vi "CANOpen_Send SDOs from list.vi"(6 "SDO queues":T1, 7 "Nodes":T4[](array[typedef]) {"NMT"."Node init static SDO state" items=["start remote node"=1, "enter pre-operational"=128]; "NMT"."Node run state" items=["start remote node"=1, "stop remote node"=2, "enter pre-operational"=128, "reset node"=129, "reset communication"=130]; "Dynamic SDOs"."Sub-Index (0)" format="%.0x"; "Dynamic SDOs"."Object Index" format="%.0x"; "Dynamic SDOs"."Block Data" format="%.0x"; "RPDOs"."PDO Channel" items=["PDO 1", "PDO 2", "PDO 3", "PDO 4"]; "RPDOs"."Parameters"."Bit Offset" max=8 step=1; "RPDOs"."Parameters"."Byte Offset" max=8 step=1; "TPDOs"."PDO Channel" items=["PDO 1", "PDO 2", "PDO 3", "PDO 4"]; "TPDOs"."Parameters"."Bit Offset" max=8 step=1; "TPDOs"."Parameters"."Byte Offset" max=8 step=1; "SDOs"."Sub-Index (0)" format="%.0x"; "SDOs"."Object Index" format="%.0x"; "SDOs"."Block Data" format="%.0x"}, 8 "error in":errorcluster, 10 "SDO Asynch":T2 {"HW Dyn Read"."Resp Chan."."Chan Refs" format="%.0x"; "HW Dyn Read"."Req Chan."."Chan Refs" format="%.0x"; "HW Dyn Write"."Resp Chan."."Chan Refs" format="%.0x"; "HW Dyn Write"."Req Chan."."Chan Refs" format="%.0x"; "List SDO"."Resp Chan."."Chan Refs" format="%.0x"; "List SDO"."Req Chan."."Chan Refs" format="%.0x"}, 11 "interface object":refnum<k20>) -> (0 "error out":errorcluster, 3 "interface object out":refnum<k20>)   [LabVIEW 2013, in "CANOpen Addon Custom Device.lvlib"]
uses:
  CANOpen Addon Custom Device.lvlib
  CANOpen_Node Message Settings.ctl
  Shared Code/CANOpen_PDO Settings.ctl
  Shared Code/CANOpen_PDO Parameter Settings.ctl
  Shared Code/CANOpen_PDO Data Type.ctl
  System Explorer/SubVIs/CANopen Byte Order.ctl
  Shared Code/CANOpen_SDO Settings.ctl
  CANOpen_NMT Settings.ctl
  Async VIs/CANOpen_Main/SubVIs/CanOpen_NMT_Config.ctl
  Async VIs/CANOpen_Main/SubVIs/CanOpen_NMT_Static detect.ctl
  CANOpen_VS SDOs Data Refs.ctl
  <vilib>/NI Veristand/Custom Device API/Data Reference.ctl
  Async VIs/CANOpen_Main/SubVIs/CanOpen_SDO Dynamic queue.ctl
  Shared Code/CANOpen_SDO queue W data.ctl
  Shared Code/CANOpen_SDO queue mode.ctl
  Shared Code/CANOpen_PDO Data Type in queue.ctl
  Async VIs/CANOpen_Main/SubVIs/CanOpen_SDO queue ref.ctl
  Async VIs/CANOpen_Main/SubVIs/SDO queue.ctl
  <vilib>/NI Veristand/Custom Device Tools/Custom Device Utility Library/RT Debug String Color Spec.ctl
  <vilib>/NI Veristand/Custom Device Tools/Custom Device Utility Library/Custom Device Utility Library.lvlib
  <vilib>/NI Veristand/Custom Device API/Custom Device API.lvlib
panel:
  # "LSB"
  # "MSB"
  # "LSB"
  # "MSB"
  # "LSB"
  # "MSB"
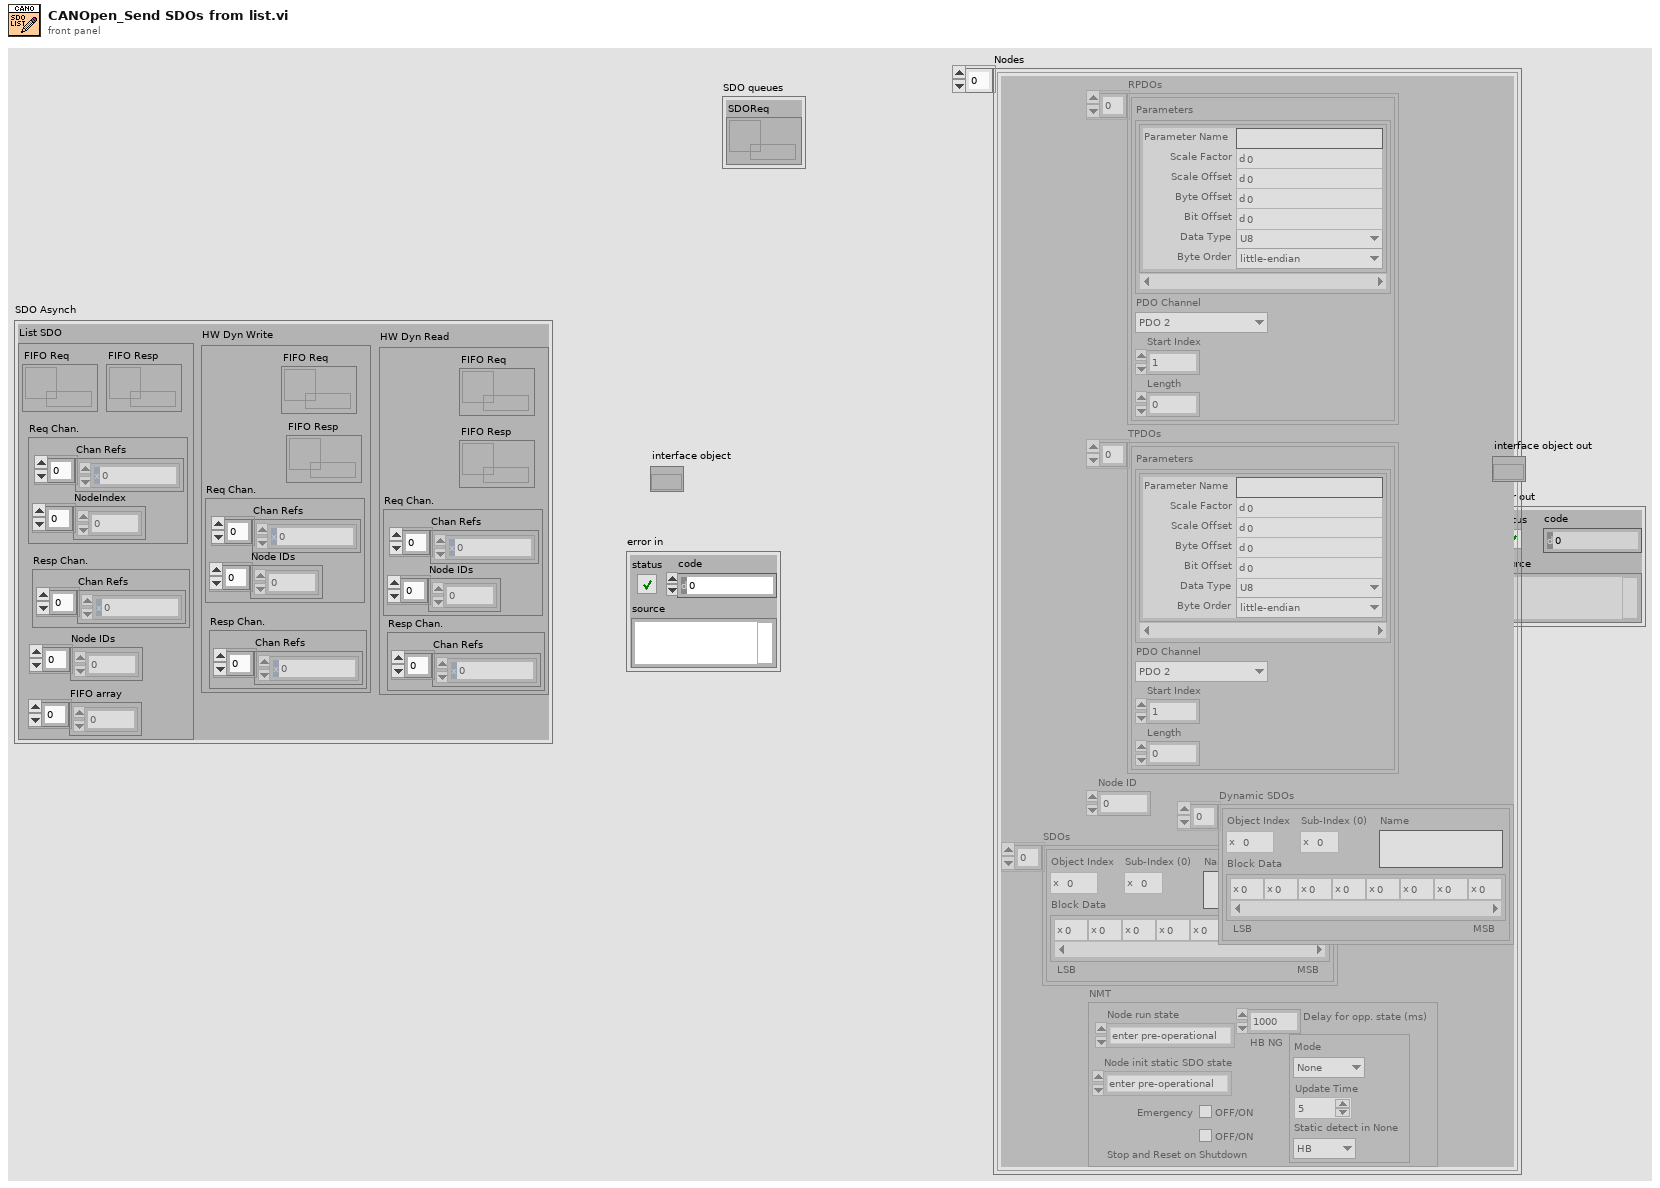
[diagram p1: front panel]
types:
  T1 = typedef "CANOpen Addon Custom Device.lvlib/CanOpen_SDO queue ref.ctl" = cluster{"SDOReq":refnum<queue>}
  T2 = typedef "CANOpen Addon Custom Device.lvlib/CANOpen_VS SDOs Data Refs.ctl" = cluster{"List SDO":cluster{"FIFO Req":refnum<k33>, "Req Chan.":cluster{"Chan Refs":T3[], "NodeIndex":dbl[]}, "FIFO Resp":refnum<k33>, "Resp Chan.":cluster{"Chan Refs":T3[]}, "Node IDs":u8[], "FIFO array":dbl[]}, "HW Dyn Write":cluster{"FIFO Req":refnum<k33>, "FIFO Resp":refnum<k33>, "Req Chan.":cluster{"Chan Refs":T3[], "Node IDs":u8[]}, "Resp Chan.":cluster{"Chan Refs":T3[]}}, "HW Dyn Read":cluster{"FIFO Req":refnum<k33>, "FIFO Resp":refnum<k33>, "Req Chan.":cluster{"Chan Refs":T3[], "Node IDs":u8[]}, "Resp Chan.":cluster{"Chan Refs":T3[]}}}
  T3 = typedef "Custom Device API.lvlib/Data Reference.ctl" = i32
  T4 = typedef "CANOpen_Node Message Settings.ctl" = cluster{"RPDOs":T5[], "TPDOs":T5[], "Node ID":u8, "SDOs":T9[], "Dynamic SDOs":T9[], "NMT":T10}
  T5 = typedef "CANOpen Addon Custom Device.lvlib/CANOpen_PDO Settings.ctl" = cluster{"Parameters":T6[], "PDO Channel":u8, "Start Index":u32, "Length":u32}
  T6 = typedef "CANOpen Addon Custom Device.lvlib/CANOpen_PDO Parameter Settings.ctl" = cluster{"Parameter Name":string, "Scale Factor":dbl, "Scale Offset":dbl, "Byte Offset":u8, "Bit Offset":u8, "Data Type":T7, "Byte Order":T8}
  T7 = typedef "CANOpen Addon Custom Device.lvlib/CANOpen_PDO Data Type.ctl" = enum16{"U8", "U16", "U32", "I8", "I16", "I32", "Single", "Double", "Boolean"}
  T8 = typedef "CANOpen Addon Custom Device.lvlib/CANopen Byte Order.ctl" = enum16{"big-endian network order", "little-endian"}
  T9 = typedef "CANOpen Addon Custom Device.lvlib/CANOpen_SDO Settings.ctl" = cluster{"Object Index":u16, "Sub-Index (0)":u8, "Block Data":u8[], "Name":string}
  T10 = typedef "CANOpen Addon Custom Device.lvlib/CANOpen_NMT Settings.ctl" = cluster{"Node run state":u16, "Emergency":bool, "HB NG":T11, "Delay for opp. state (ms)":dbl, "Node init static SDO state":u16, "Stop and Reset on Shutdown":bool}
  T11 = typedef "CANOpen Addon Custom Device.lvlib/CanOpen_NMT_Config.ctl" = cluster{"Mode":T12, "Update Time":u16, "Static detect in None":T12}
  T12 = typedef "CANOpen Addon Custom Device.lvlib/CanOpen_NMT_Static detect.ctl" = enum16{"None", "HB", "NG"}
  T13 = typedef "CANOpen Addon Custom Device.lvlib/CanOpen_SDO Dynamic queue.ctl" = cluster{"Node ID":u8, "Data":T14}
  T14 = typedef "CANOpen Addon Custom Device.lvlib/CANOpen_SDO queue W data.ctl" = cluster{"Object Index":u16, "Object Sub-Index (0)":u8, "Mode":T15, "Data Type":T16, "Value":dbl, "Status code":dbl, "Byte Order":enum16{"big-endian, network order", "little-endian"}}
  T15 = typedef "CANOpen Addon Custom Device.lvlib/CANOpen_SDO queue mode.ctl" = enum16{"WRITE write", "WRITE response", "READ write", "READ response"}
  T16 = typedef "CANOpen Addon Custom Device.lvlib/CANOpen_PDO Data Type in queue.ctl" = enum16{"U8", "U16", "U32", "I8", "I16", "I32", "Single", "Double"}
  T17 = typedef "CANOpen Addon Custom Device.lvlib/SDO queue.ctl" = cluster{"element":T9, "Node ID":u8}
  T18 = typedef "Custom Device Utility Library.lvlib/RT Debug String Color Spec.ctl" = u16
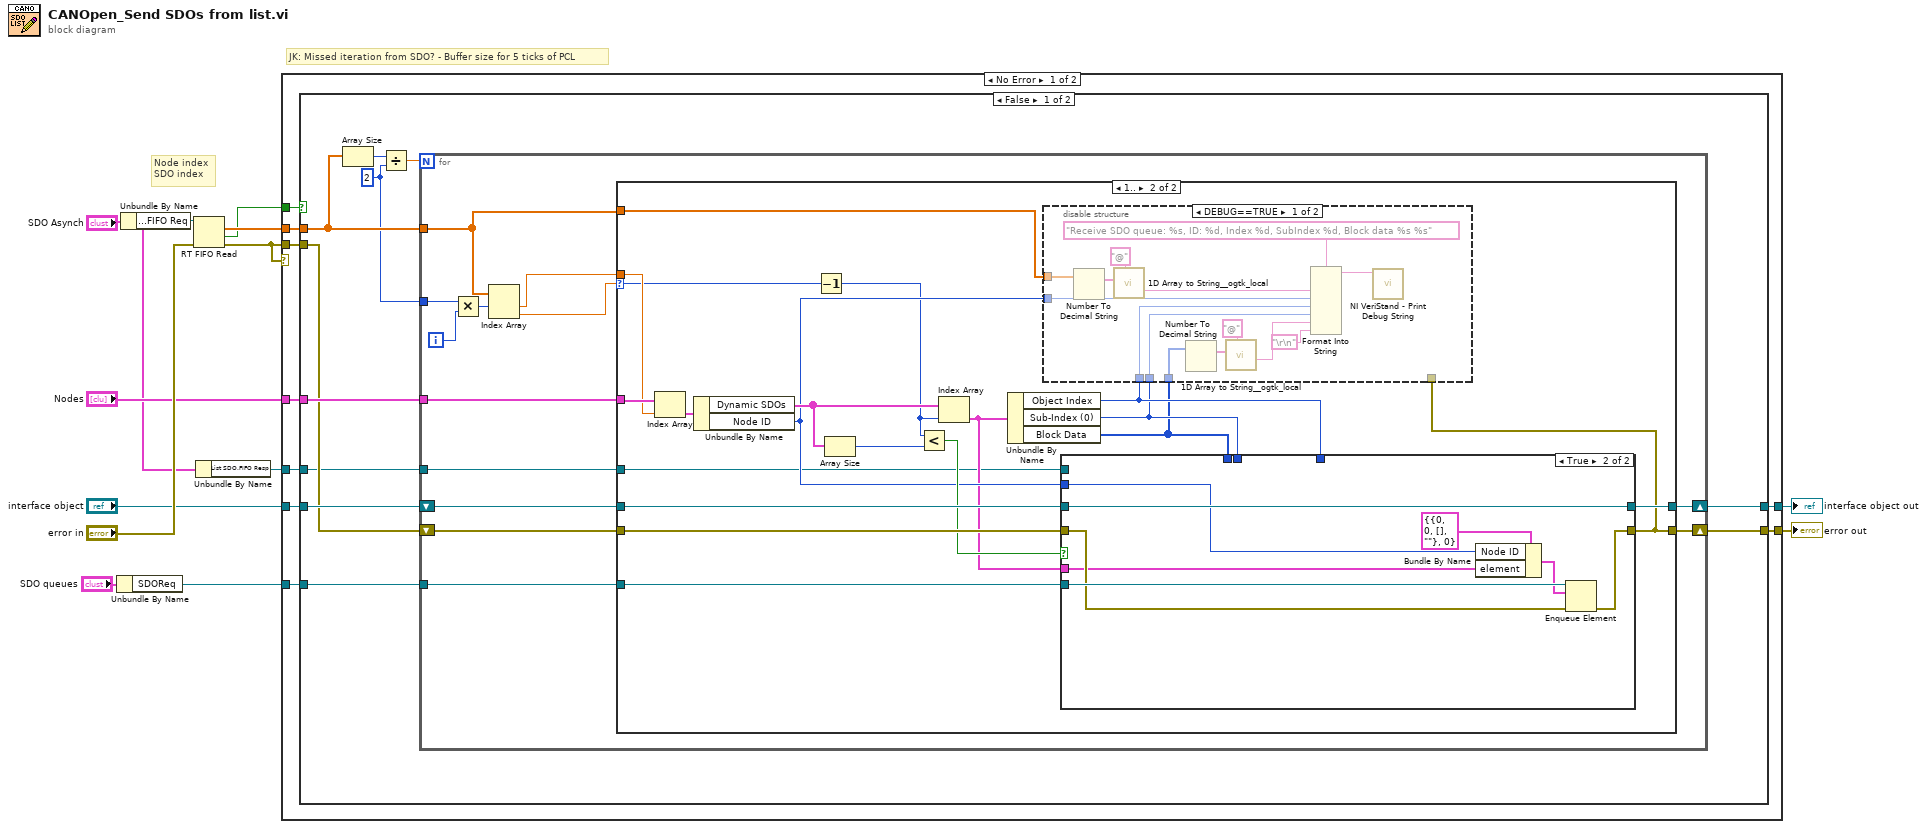
[diagram p0: block diagram]
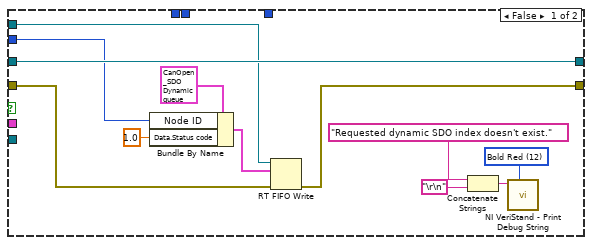
[diagram p3: hidden frame]
diagram:
  # "Node index\nSDO index"
  # "JK: Missed iteration from SDO? - Buffer size for 5 ticks of PCL"
  n1 = Unbundle By Name("SDO queues") -> ("SDOReq"=w5:refnum<queue>)
  n2 = Unbundle By Name("SDO Asynch") -> ("List SDO.FIFO Req"=w4:refnum<k33>)
  n3 = RT FIFO Read(0:w4, 3:"error in") -> (9:w8:dbl[], 10:w7:bool, 11:w3:errorcluster)  [unwired: 2 in, 2 out]
  n4 = Unbundle By Name("SDO Asynch") -> ("List SDO.FIFO Resp"=w1:refnum<k33>)
  n5 = case shown="No Error" w3 {
    tunnel: "Nodes" -> [w22 _]
    tunnel: "interface object" -> [w21 w106]
    tunnel: w3 -> [w20 w105]
    tunnel: [w19 w105] -> w10
    tunnel: [w18 w106] -> w9
    tunnel: w8 -> [w17 _]
    tunnel: w7 -> [w16 _]
    tunnel: w5 -> [w15 _]
    tunnel: w1 -> [w14 _]
    frame No Error {
      n6 = case shown="False" w16 {
        tunnel: w22 -> [w33 _]
        tunnel: w21 -> [w32 w104]
        tunnel: w20 -> [w31 w103]
        tunnel: [w30 w103] -> w19
        tunnel: [w29 w104] -> w18
        tunnel: w17 -> [w25 _]
        tunnel: w15 -> [w28 _]
        tunnel: w14 -> [w23 _]
        frame False {
          w24 = 2 ("y")
          n7 = Array Size(array=w25) -> (size(s)=w27:i32)
          n8 = Divide(x=w27, y=w24) -> (x/y=w26:dbl)
          n9 = for {
            N: w26 -> [_]
            tunnel: w33 -> [w46]
            tunnel: w25 -> [w38]
            tunnel: w28 -> [w41]
            shift-right: [w42] -> w29
            shift-left: w32 -> [w45]
            shift-right: [w43] -> w30
            shift-left: w31 -> [w44]
            tunnel: w24 -> [w36]
            tunnel: w23 -> [w34]
            i -> [w37]
            n10 = Multiply(x=w36, y=w37) -> (x*y=w40:i32)
            n11 = Index Array(array=w38, index #1=w40) -> (element #1=w39:dbl, element #2=w35:dbl)  [unwired: 1 in]
            n12 = case shown="1.." w35 {
              selector: w35 -> [_ w60]
              tunnel: w46 -> [_ w68]
              tunnel: w39 -> [_ w67]
              tunnel: w45 -> [w48 w65]
              tunnel: w44 -> [w47 w64]
              tunnel: [w47 w52] -> w43
              tunnel: [w48 w63] -> w42
              tunnel: w38 -> [_ w62]
              tunnel: w41 -> [_ w50]
              tunnel: w34 -> [_ w49]
              frame 0, Default {
              }
              frame 1.. {
                n13 = Index Array(array=w68, index=w67) -> (element=w66:T4)
                n14 = Unbundle By Name(w66) -> ("Dynamic SDOs"=w61:T9[], "Node ID"=w57:u8)
                n15 = Decrement(x=w60) -> (x-1=w53:i32)
                n16 = Array Size(array=w61) -> (size(s)=w59:i32)
                n17 = Less?(x=w53, y=w59) -> (x < y?=w58:bool)
                n18 = Index Array(array=w61, index=w53) -> (element=w51:T9)
                n19 = Unbundle By Name(w51) -> ("Object Index"=w56:u16, "Sub-Index (0)"=w55:u8, "Block Data"=w54:u8[])
                n20 = case shown="True" w58 {
                  tunnel: w65 -> [w80 w88]
                  tunnel: w64 -> [w71 w85]
                  tunnel: [w80 w88] -> w63
                  tunnel: [w70 w83] -> w52
                  tunnel: w56 -> [_ _]
                  tunnel: w55 -> [_ _]
                  tunnel: w54 -> [_ _]
                  tunnel: w57 -> [w73 w81]
                  tunnel: w51 -> [_ w84]
                  tunnel: w50 -> [_ w86]
                  tunnel: w49 -> [w72 _]
                  frame False {
                    w76 = T18 12 items=["Plain White"=7, "Bold White"=15, "Bold Blue"=9, "Bold Green"=10, "Bold Red"=12] ("Attribute")
                    n21 = Bundle By Name(cluster=T13 {"Node ID"=0, "Data"={"Object Index"=0, "Object Sub-Index (0)"=0, "Mode"=enum."WRITE response", "Data Type"=enum."Double", "Value"=0.0, "Status code"=0.0, "Byte Order"=enum."big-endian, network order"}} ("element"), "Node ID"=w73, "Data.Status code"=1.0) -> (w74:T13)
                    n22 = RT FIFO Write(0:w72, 1:w74, 3:w71) -> (11:w70:errorcluster)  [unwired: 2 in, 3 out]
                    n23 = Concatenate Strings("Requested dynamic SDO index doesn't exist." ("string"), "\r\n") -> (w79:string)
                    n24 = call <vilib>:"NI VeriStand - Print Debug String.vi"("Attribute"=w76, "Message"=w79) -> ()  [unwired: 9 in, 1 out]
                  }
                  frame True {
                    n25 = Bundle By Name(cluster=T17 {"element"={"Object Index"=0, "Sub-Index (0)"=0, "Block Data"=[], "Name"=""}, "Node ID"=0} ("Cluster"), "Node ID"=w81, "element"=w84) -> (w82:T17)
                    n26 = Enqueue Element(queue=w86, element=w82, error in (no error)=w85) -> (error out=w83:errorcluster)  [unwired: 1 in, 2 out]
                  }
                }
                n27 = disable-structure shown="DEBUG==TRUE" {
                  disable-tunnel: w62 -> [w100 _]
                  disable-tunnel: w57 -> [w96 _]
                  disable-tunnel: w56 -> [w95 _]
                  disable-tunnel: w55 -> [w94 _]
                  disable-tunnel: w54 -> [w91 _]
                  disable-tunnel: w52 -> [_ _]
                  frame condition #0 {
                    n28 = Number To Decimal String(number=w100) -> (decimal integer string=w101:string[])  [unwired: 1 in]
                    n29 = call "1D Array to String__ogtk_local.vi"("delimiter (Tab)"="@", "Array of Strings"=w101) -> ("delimited string"=w97:string)  [unwired: 9 in]
                    n30 = Number To Decimal String(number=w91) -> (decimal integer string=w92:string[])  [unwired: 1 in]
                    n31 = call "1D Array to String__ogtk_local.vi"("delimiter (Tab)"="@", "Array of Strings"=w92) -> ("delimited string"=w90:string)  [unwired: 9 in]
                    n32 = Format Into String(format string="Receive SDO queue: %s, ID: %d, Index %d, SubIndex %d, Block data %s %s", w97, w96, w95, w94, w90, "\r\n") -> (resulting string=w98:string)  [unwired: 2 in, 1 out]
                    n33 = call <vilib>:"NI VeriStand - Print Debug String.vi"("Message"=w98) -> ()  [unwired: 10 in, 1 out]
                  }
                  frame condition #1 (active) {
                  }
                }
              }
            }
          }
        }
        frame True {
        }
      }
    }
    frame Error {
    }
  }
  "error out" <- w10
  "interface object out" <- w9
